vi "LED_Execute.vi"() -> ()   [LabVIEW 2019]
uses:
  LED_States.ctl
  Globals/LED_Globals.vi
panel:
  in  "blink_delay":u32
  in  "LED_States":T1
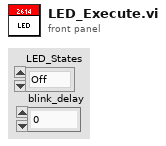
[diagram p1: front panel]
types:
  T1 = typedef "LED_States.ctl" = enum16{"Off", "Red", "Green", "Yellow", "Blue", "Purple", "Turqoise", "White", "Off Blinking", "Red Blinking", "Green Blinking", "Yellow Blinking", "Blue Blinking", "Purple Blinking", "Turqoise Blinking", "White Blinking"}
  T2 = typedef "CTRE_CANifier_DeviceRef.ctl" = cluster{"DeviceStatus":errorcluster, "Device Number":u8, "Handle":u64, "UsageFrame":u32, "Library Path":path}
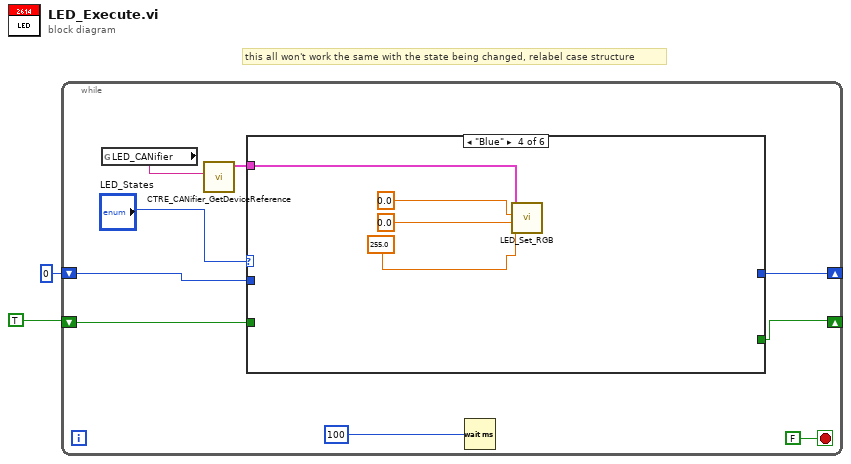
[diagram p0: block diagram]
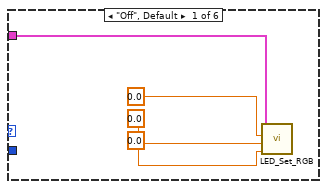
[diagram p2: hidden frame]
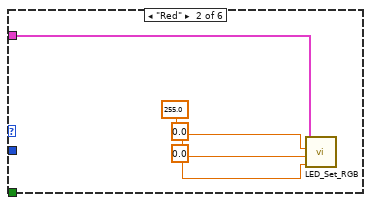
[diagram p3: hidden frame]
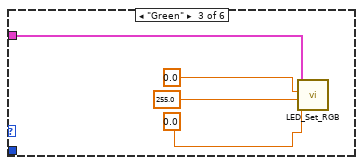
[diagram p4: hidden frame]
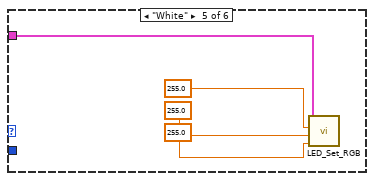
[diagram p5: hidden frame]
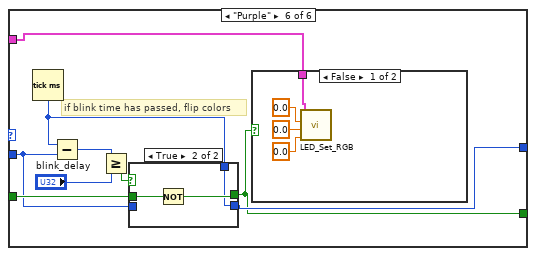
[diagram p6: hidden frame]
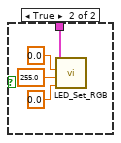
[diagram p8: hidden frame]
diagram:
  # "this all won't work the same with the state being changed, relabel case structure"
  n1 = while {
    shift-right: [w3] -> _
    shift-left: TRUE -> [w6]
    shift-right: [w5] -> _
    shift-left: u32 0 ("blink_delay") -> [w4]
    stop <- FALSE stop-if-true
    n2 = global read "LED_Globals.vi" "LED_CANifier"() -> (w9:string)
    n3 = call <vilib>:"CTRE_CANifier_GetDeviceReference.vi"("refnum name"=w9) -> ("CANifierDevRef"=w8:T2)  [unwired: 9 in, 1 out]
    n4 = case shown="\"Blue\"" "LED_States" {
      tunnel: w8 -> [w15 w16 w20 w24 w28 w40]
      tunnel: w6 -> [_ _ _ _ _ w36]
      tunnel: [_ _ _ _ _ w35] -> w5
      tunnel: w4 -> [_ _ _ _ _ w34]
      tunnel: [_ _ _ _ _ w32] -> w3
      frame "Off", Default {
        n5 = call "LED_Set_RGB.vi"("B"=0.0, "G"=0.0, "R"=0.0, "CANifierDevRef"=w15) -> ()  [unwired: 8 in]
      }
      frame "Red" {
        n6 = call "LED_Set_RGB.vi"("B"=0.0, "G"=0.0, "R"=255.0, "CANifierDevRef"=w16) -> ()  [unwired: 8 in]
      }
      frame "Green" {
        n7 = call "LED_Set_RGB.vi"("B"=0.0, "G"=255.0, "R"=0.0, "CANifierDevRef"=w20) -> ()  [unwired: 8 in]
      }
      frame "Blue" {
        n8 = call "LED_Set_RGB.vi"("B"=255.0, "G"=0.0, "R"=0.0, "CANifierDevRef"=w24) -> ()  [unwired: 8 in]
      }
      frame "White" {
        n9 = call "LED_Set_RGB.vi"("B"=255.0, "G"=255.0, "R"=255.0, "CANifierDevRef"=w28) -> ()  [unwired: 8 in]
      }
      frame "Purple" {
        # "if blink time has passed, flip colors"
        n10 = Tick Count (ms)() -> (millisecond timer value=w33:u32)
        n11 = Subtract(x=w33, y=w34) -> (x-y=w39:u32)
        n12 = Greater Or Equal?(x=w39, y="blink_delay") -> (x >= y?=w37:bool)
        n13 = case shown="True" w37 {
          tunnel: [w41 w44] -> w32
          tunnel: w36 -> [w41 w45]
          tunnel: [w42 w43] -> w35
          tunnel: w34 -> [w42 _]
          tunnel: w33 -> [_ w43]
          frame False {
          }
          frame True {
            n14 = Not(x=w45) -> (.not. x?=w44:bool)
          }
        }
        n15 = case shown="False" w32 {
          tunnel: w40 -> [w46 w50]
          frame False {
            n16 = call "LED_Set_RGB.vi"("B"=0.0, "G"=0.0, "R"=0.0, "CANifierDevRef"=w46) -> ()  [unwired: 8 in]
          }
          frame True {
            n17 = call "LED_Set_RGB.vi"("B"=0.0, "G"=255.0, "R"=0.0, "CANifierDevRef"=w50) -> ()  [unwired: 8 in]
          }
        }
      }
    }
    n18 = Wait (ms)(milliseconds to wait=u32 100) -> ()  [unwired: 1 out]
  }
